vi "rename channel.vi"(8 "error in":errorcluster, 9 "new name":string, 10 "old name":string, 11 "alarms module configuration in":refnum<class "tag select module configuration.lvclass">=refnum) -> (0 "error out":errorcluster, 3 "alarms module configuration out":refnum<class "tag select module configuration.lvclass">)   [LabVIEW 2013]
uses:
  <vilib>/NI/Tag Bus/tag/tag descriptor.lvclass
  tag select module configuration.lvclass
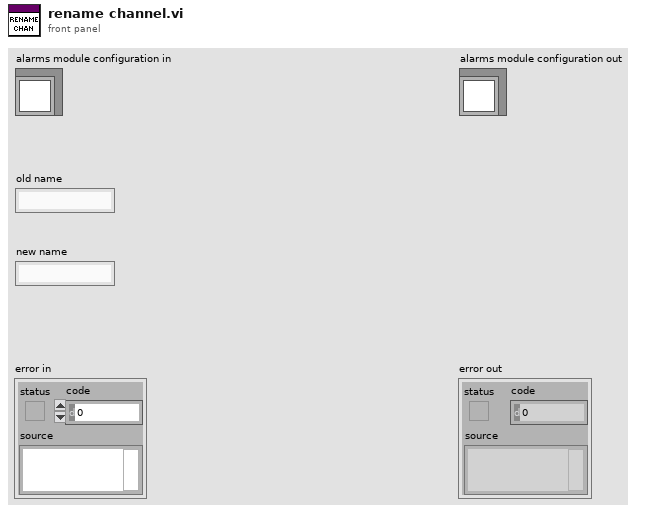
[diagram p1: front panel]
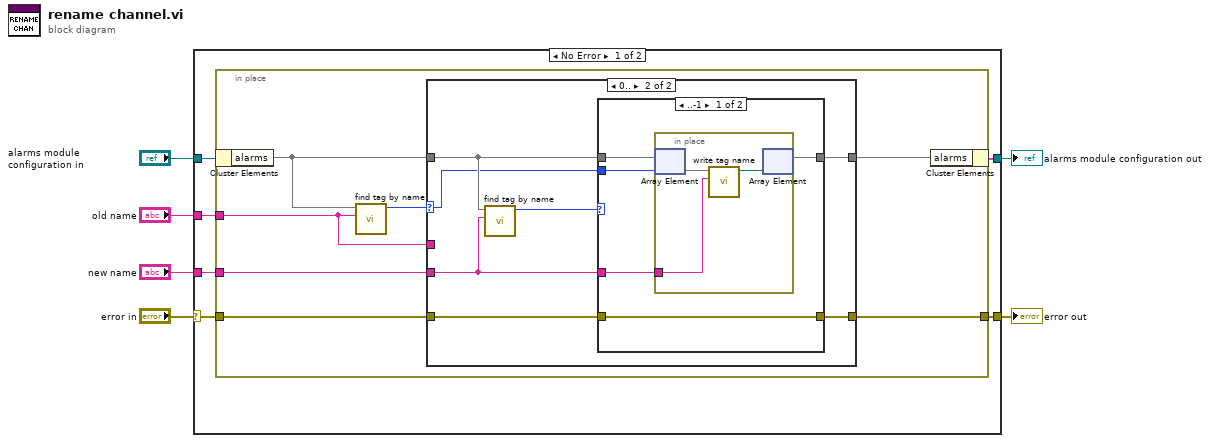
[diagram p0: block diagram]
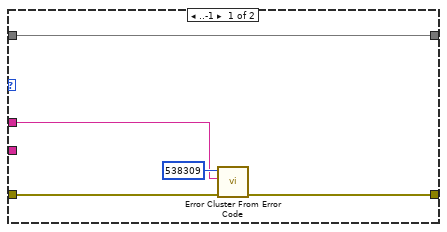
[diagram p2: hidden frame]
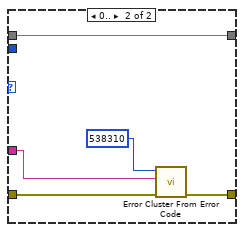
[diagram p3: hidden frame]
diagram:
  n1 = case shown="No Error" "error in" {
    selector: "error in" -> [w7 w46]
    tunnel: "new name" -> [w12 _]
    tunnel: "alarms module configuration in" -> [w11 w45]
    tunnel: [w10 w45] -> w4
    tunnel: [w9 w46] -> w3
    tunnel: "old name" -> [w8 _]
    frame No Error {
      n2 = in-place {
        in-place-border: w8 -> [w18]
        in-place-border: w12 -> [w14]
        in-place-border: [w17] -> w9
        in-place-border: w7 -> [w15]
        n3 = in-place-cluster #1(w11) -> ("alarms"=w19)
        n4 = call <vilib>:"find tag by name.vi"("name"=w18, "tags in"=w19) -> ("index"=w13:i32)  [unwired: 9 in]
        n5 = case shown="0.." w13 {
          selector: w13 -> [_ w25]
          tunnel: w19 -> [w21 w30]
          tunnel: w18 -> [w23 _]
          tunnel: [w22 w26] -> w17
          tunnel: [w21 w31] -> w16
          tunnel: w15 -> [w20 w27]
          tunnel: w14 -> [_ w29]
          frame ..-1 {
            n6 = call <vilib>:"Error Cluster From Error Code.vi"("error in (no error)"=w20, "error message (\"\")"=w23, "error code (0)"=538309) -> ("error out"=w22:errorcluster)  [unwired: 6 in]
          }
          frame 0.. {
            n7 = call <vilib>:"find tag by name.vi"("name"=w29, "tags in"=w30) -> ("index"=w28:i32)  [unwired: 9 in]
            n8 = case shown="..-1" w28 {
              tunnel: [w36 w44] -> w31
              tunnel: w25 -> [w35 _]
              tunnel: w30 -> [w34 w44]
              tunnel: w29 -> [w33 w40]
              tunnel: w27 -> [w32 w42]
              tunnel: [w32 w43] -> w26
              frame ..-1 {
                n9 = in-place {
                  in-place-border: w33 -> [w37]
                  n10 = in-place-array #2(w34, w35) -> (w39)
                  n11 = call <vilib>:"write tag name.vi"("name"=w37, "system tag in"=w39) -> ("system tag out"=w38:refnum<class "tag descriptor.lvclass">)  [unwired: 8 in, 1 out]
                  n12 = in-place-array #2(w38) -> (w36)  [unwired: 1 out]
                }
              }
              frame 0.. {
                n13 = call <vilib>:"Error Cluster From Error Code.vi"("error in (no error)"=w42, "error message (\"\")"=w40, "error code (0)"=538310) -> ("error out"=w43:errorcluster)  [unwired: 6 in]
              }
            }
          }
        }
        n14 = in-place-cluster #1("alarms"=w16) -> (w10:cluster{})
      }
    }
    frame Error {
    }
  }
  "error out" <- w3
  "alarms module configuration out" <- w4
